vi "Reset.vi"(8 "error in (no error)":errorcluster, 10 "Message in":refnum<class "ResetMessage.lvclass">, 11 "LineCCD in":refnum<class "LineCCD.lvclass">) -> (0 "error out":errorcluster, 3 "LineCCD out":refnum<class "LineCCD.lvclass">)   [LabVIEW 2012, in "LineCCD.lvclass"]
doc: "The reset method processes the command 'reset'. \n\nResets the internal state of the component (without performing a full initialisation). This could be resetting hardware, or private data to default values."
uses:
  LineCCD.lvclass
  <vilib>/Distrio/Murmex/Murmex/Murmex.lvclass
  <vilib>/Distrio/Murmex/ResetMessage/ResetMessage.lvclass
panel:
  # "This method is called when the RESET\ntrigger is sent. \n\nOverride this method when your component needs to\nrespond to this trigger. \n\nCall parent for proper implementation"
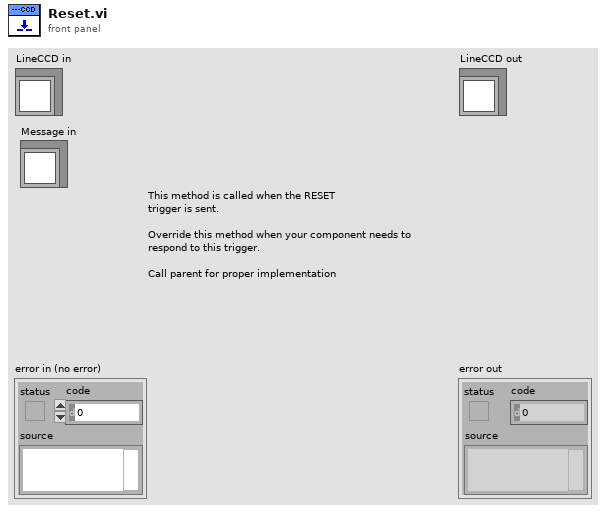
[diagram p1: front panel]
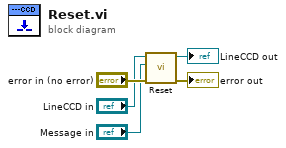
[diagram p0: block diagram]
diagram:
  n1 = call-parent "Reset.vi"("error in (no error)"="error in (no error)", "Message in"="Message in", "Murmex in"="LineCCD in") -> ("error out"=→"error out":errorcluster, "Murmex out"=→"LineCCD out":refnum<class "LineCCD.lvclass">)  [unwired: 7 in]
